vi "Battery_monitor.vi"() -> ()   [LabVIEW 2020]
uses:
  States_enum.ctl
  <vilib>/Utility/config.llb/Read Key (String).vi
  <vilib>/Utility/config.llb/Write Key (String).vi
  <vilib>/Utility/config.llb/Read Key (U32).vi
  <vilib>/Utility/config.llb/Write Key (U32).vi
  <vilib>/Utility/config.llb/NI_LVConfig.lvlib
panel:
  out "IP address:":string
  out "Enum":T1
  in  "stop":bool
  out "Tab Control":enum32{"Page 1", "Page 2"}(tab)
  out "output cluster":T2
  in  "init":bool
  out "input cluster":T3
  out "error out":errorcluster
  out "Connection configuration 2":T2
  out "connection ID":refnum<k5>
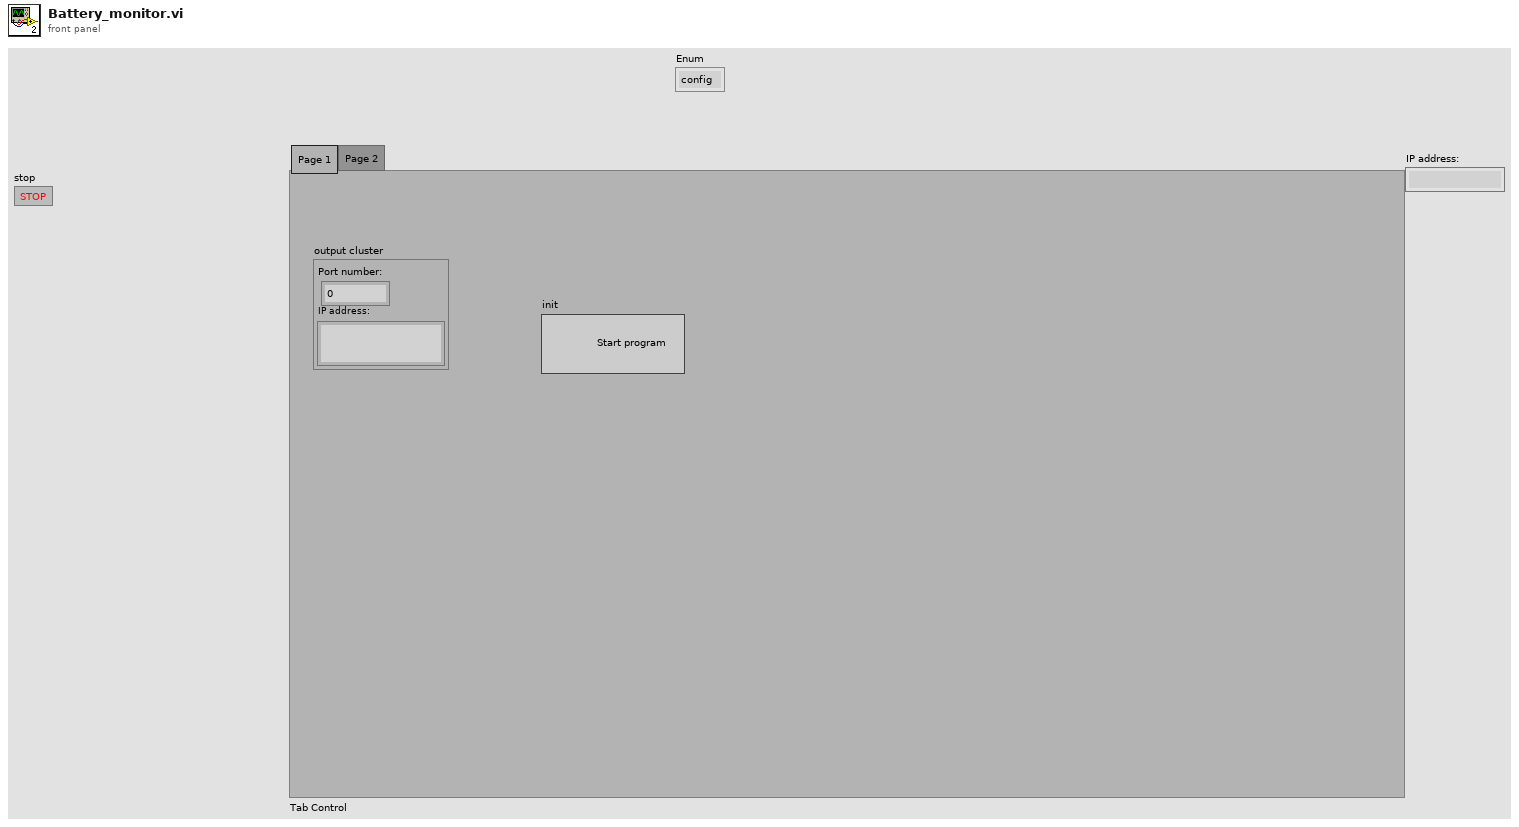
[diagram p1: front panel]
types:
  T1 = typedef "States_enum.ctl" = enum16{"config", "init", "monitor", "stop"}
  T2 = cluster{"Port number:":u32, "IP address:":string}
  T3 = cluster{"time":timestamp, "voltage":dbl, "genarator_running":bool, "aux_on":bool, "alarm":bool, "low_fuel":bool}
  T4 = typedef "NI_LVConfig.lvlib/Config Data RefNum.ctl" = refnum<k1>
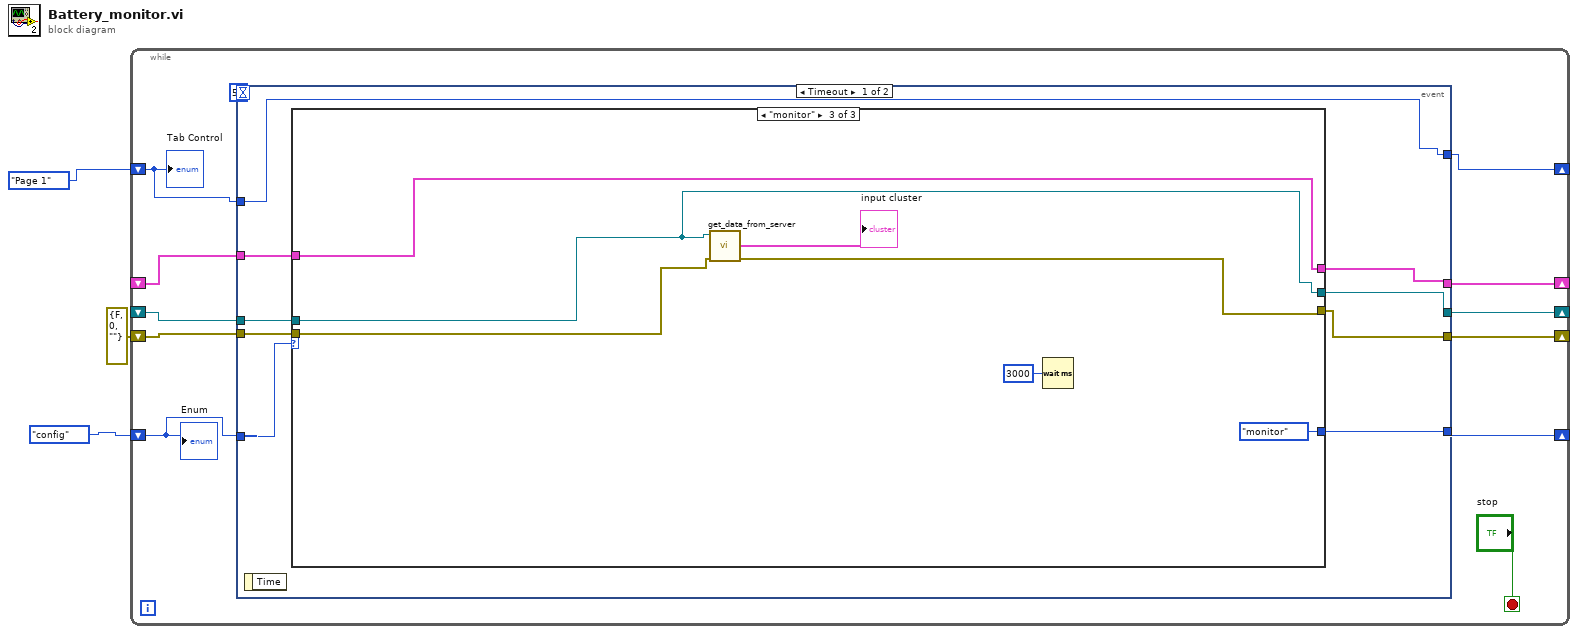
[diagram p0: block diagram]
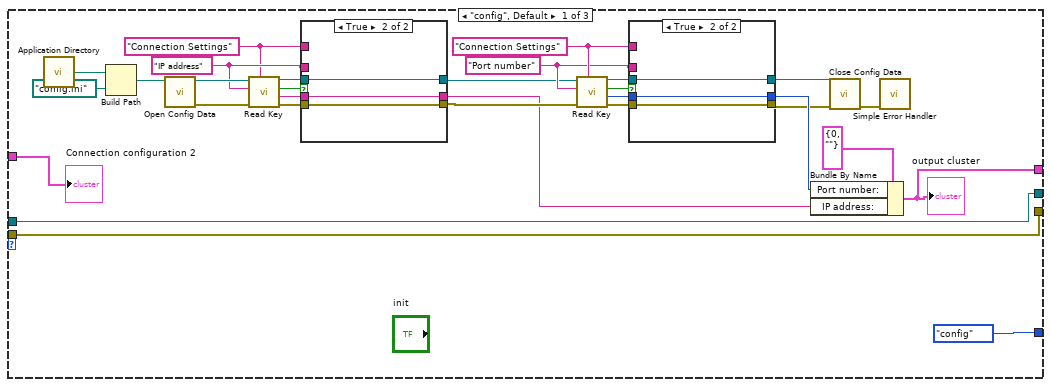
[diagram p2: hidden frame]
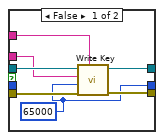
[diagram p3: hidden frame]
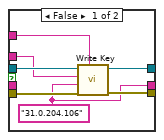
[diagram p4: hidden frame]
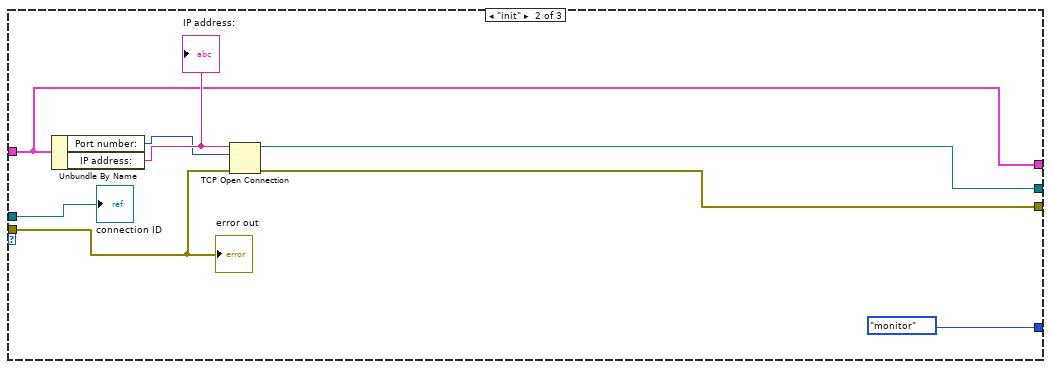
[diagram p5: hidden frame]
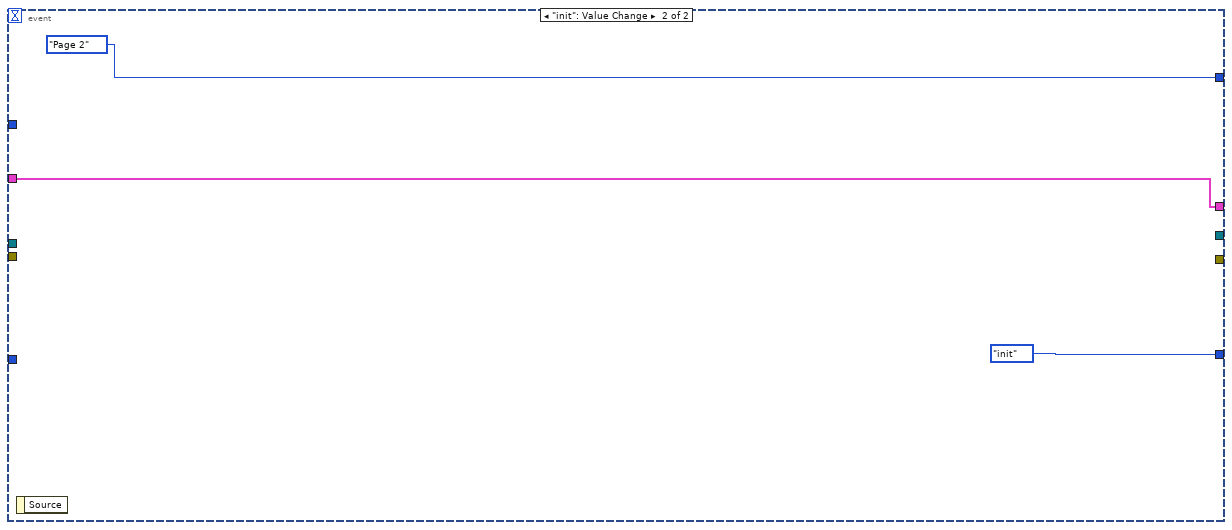
[diagram p6: hidden frame]
diagram:
  n1 = while {
    shift-right: [w12] -> _
    shift-left: States_enum."config" -> [w13]
    shift-right: [w11] -> _
    shift-left: _ -> [w10]
    shift-right: [w9] -> _
    shift-left: _ -> [w8]
    shift-right: [w7] -> _
    shift-left: errorcluster {"status"=FALSE, "code"=0, "source"=""} ("error out") -> [w6]
    shift-right: [w5] -> _
    shift-left: enum32{"Page 1", "Page 2"}."Page 1" ("Tab Control") -> [w4]
    stop <- "stop" stop-if-true
    n2 = event shown="[0] Timeout" {
      selector: _ -> [_ _]
      dyn-events: _ -> [_ _]
      timeout: 50 -> [_ _]
      tunnel: w13 -> [w24 _]
      tunnel: [w23 States_enum."init"] -> w12
      tunnel: [w22 w91] -> w11
      tunnel: w10 -> [w21 w91]
      tunnel: [w20 _] -> w9
      tunnel: w8 -> [w19 _]
      tunnel: [w18 _] -> w7
      tunnel: w6 -> [w17 _]
      tunnel: [w16 enum32{"Page 1", "Page 2"}."Page 2" ("Tab Control 2")] -> w5
      tunnel: w4 -> [w16 _]
      event Timeout {
        n3 = event-data() -> ()  [unwired: 1 in, 1 out]
        n4 = case shown="\"monitor\"" w24 {
          tunnel: [States_enum."config" States_enum."monitor" States_enum."monitor"] -> w23
          tunnel: [w28 w79 w89] -> w22
          tunnel: w21 -> [w25 w79 w89]
          tunnel: [w26 w78 w85] -> w20
          tunnel: w19 -> [w26 w76 w85]
          tunnel: [w27 w77 w86] -> w18
          tunnel: w17 -> [w27 w75 w87]
          frame "config", Default {
            w39 = "Port number" ("key")
            w40 = "Connection Settings" ("section")
            w48 = "IP address" ("key")
            w47 = "Connection Settings" ("section")
            n5 = call <vilib>:"Application Directory.vi"() -> ("Application Directory"=w54:path)
            n6 = Build Path(base path=w54, name or relative path=path "config.ini") -> (appended path=w52:path)
            n7 = call <vilib>:"Open Config Data.vi"("configuration file path"=w52) -> ("error out"=w51:errorcluster, "refnum"=w50:T4)  [unwired: 8 in, 1 out]
            n8 = call-poly <vilib>:"Read Key.vi"("section"=w47, "error in (no error)"=w51, "key"=w48, "refnum"=w50) -> ("error out"=w45:errorcluster, "value"=w44:string, "found?"=w46:bool, "refnum out"=w49:T4)  [unwired: 4 in]
            n9 = case shown="True" w46 {
              tunnel: w49 -> [w71 w74]
              tunnel: w48 -> [w70 _]
              tunnel: w47 -> [w69 _]
              tunnel: w45 -> [w68 w73]
              tunnel: [w67 w73] -> w37
              tunnel: [w66 w74] -> w36
              tunnel: w44 -> [_ w72]
              tunnel: [w65 w72] -> w35
              frame False {
                w65 = "31.0.204.106"
                n10 = call-poly <vilib>:"Write Key.vi"("section"=w69, "error in (no error)"=w68, "value"=w65, "key"=w70, "refnum"=w71) -> ("error out"=w67:errorcluster, "refnum out"=w66:T4)  [unwired: 4 in, 1 out]
              }
              frame True {
              }
            }
            n11 = call-poly <vilib>:"Read Key.vi"("section"=w40, "error in (no error)"=w37, "key"=w39, "refnum"=w36) -> ("error out"=w42:errorcluster, "value"=w43:u32, "found?"=w41:bool, "refnum out"=w38:T4)  [unwired: 4 in]
            n12 = case shown="True" w41 {
              tunnel: w38 -> [w61 w64]
              tunnel: w39 -> [w60 _]
              tunnel: w40 -> [w59 _]
              tunnel: w42 -> [w58 w63]
              tunnel: [w57 w63] -> w33
              tunnel: [w56 w64] -> w32
              tunnel: w43 -> [_ w62]
              tunnel: [w55 w62] -> w34
              frame False {
                w55 = u32 65000
                n13 = call-poly <vilib>:"Write Key.vi"("section"=w59, "error in (no error)"=w58, "value"=w55, "key"=w60, "refnum"=w61) -> ("error out"=w57:errorcluster, "refnum out"=w56:T4)  [unwired: 4 in, 1 out]
              }
              frame True {
              }
            }
            n14 = Bundle By Name(cluster=T2 {"Port number:"=0, "IP address:"=""} ("Connection configuration 2"), "Port number:"=w34, "IP address:"=w35) -> (w28:T2)
            "output cluster" <- w28
            n15 = call <vilib>:"Close Config Data.vi"("error in (no error)"=w33, "refnum"=w32) -> ("error out"=w31:errorcluster)  [unwired: 8 in, 1 out]
            n16 = call <vilib>:"Simple Error Handler.vi"("error in (no error)"=w31) -> ()  [unwired: 4 in, 5 out]
            "Connection configuration 2" <- w25
          }
          frame "init" {
            n17 = Unbundle By Name(w79) -> ("Port number:"=w80:u32, "IP address:"=w81:string)
            "IP address:" <- w81
            n18 = TCP Open Connection(address=w81, remote port or service name=w80, error in (no error)=w75) -> (connection ID=w78:refnum<k5>, error out=w77:errorcluster)  [unwired: 2 in]
            "error out" <- w75
            "connection ID" <- w76
          }
          frame "monitor" {
            n19 = call "get_data_from_server.vi"("error in (no error)"=w87, "TCP Network Connection in"=w85) -> ("error out"=w86:errorcluster, "input cluster"=→"input cluster":T3)  [unwired: 7 in, 1 out]
            n20 = Wait (ms)(milliseconds to wait=u32 3000) -> ()  [unwired: 1 out]
          }
        }
      }
      event "init": Value Change {
        n21 = event-data() -> ()  [unwired: 1 in, 1 out]
      }
    }
    "Enum" <- w13
    "Tab Control" <- w4
  }
